vi "FPGA_Main.vi"() -> ()   [LabVIEW 2019]
uses:
  L298N_Driver/L298N_Action_Enum.ctl
  L298N_Ref_FPGA.ctl
  <vilib>/Platform/TimedLoop/XDataNode/timing_clust.ctl
  <vilib>/Platform/TimedLoop/XDataNode/nitl_modes.ctl
  <vilib>/Platform/TimedLoop/XDataNode/wakeup.ctl
  <vilib>/rvi/Emulation/niFpgaSctlEmulationGetInTimedLoop.vi
  <vilib>/rvi/Emulation/niFpgaEmulationReportErrorSimple.vi
  <vilib>/rvi/Emulation/niFpgaGetClockAttributes.vi
  <vilib>/rvi/Emulation/niFpgaCriticalErrorInLSC.vi
  <vilib>/rvi/Emulation/niFpgaProcessEmulError.vi
  <vilib>/rvi/eio/common/nirviEmuTemplateMethod_errors.vi
  <vilib>/Platform/TimedLoop/XDataNode/XDataNode.xnode
  <vilib>/eio/EIONode/EIONode.xnode
  <vilib>/Platform/TimedLoop/XDataNode/XDNodeRunTimeDep.lvlib
panel:
  out "Presence_Cabine":bool[](array[boolean])
  out "Portes_Fermees":bool[](array[boolean])
  out "Portes_Ouvertes":bool[](array[boolean])
  in  "CMD_Moteur_Porte_3":T1
  in  "CMD_Moteur_Porte_2":T1
  in  "CMD_Moteur_Porte_1":T1
  in  "CMD_Moteur_Porte_RDC":T1
  in  "STOP":bool
  in  "CMD_Moteur_Cabine":T1
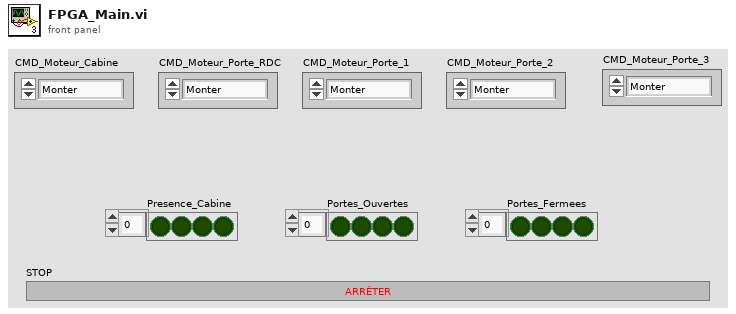
[diagram p1: front panel]
types:
  T1 = typedef "L298N_Action_Enum.ctl" = enum16{"Monter", "Descendre", "Arreter"}
  T2 = typedef "L298N_Ref_FPGA.ctl" = cluster{"Positive_Move":refnum<k21>, "Negative_Move":refnum<k21>}
  T3 = typedef "XDNodeRunTimeDep.lvlib/timing_clust.ctl" = cluster{"Expected End [f-1]":u64, "Actual End [f-1]":u64, "Finished Late? [f-1]":bool, "Expected End [i-1]":u64, "Actual End [i-1]":u64, "Finished Late? [i-1]":bool, "Expected Start [i]":u64, "Actual Start [i]":u64, "Expected Start [f]":u64, "Actual Start [f]":u64, "Source Name":string, "Structure Name":string, "Period":i64, "Deadline":i64, "Offset":i64, "Start":i64, "Priority":i32, "Timeout":i32, "Mode":T4, "Wakeup Reason":T5, "Error":errorcluster, "Source Type":string, "Secondary Source Type":string, "Global End Time":u64, "Global Start Time":u64, "Frame Duration":u64, "Iteration Duration":u64, "Assigned CPU":i32, "I/O Scan Engine Mode":u32}
  T4 = typedef "XDNodeRunTimeDep.lvlib/nitl_modes.ctl" = enum32{"No Change", "Process missed periods, maintain original phase", "Discard missed periods, maintain original phase", "Process missed periods, ignore original phase", "Discard missed periods, ignore original phase"}
  T5 = typedef "XDNodeRunTimeDep.lvlib/wakeup.ctl" = enum32{"Normal", "Aborted", "Asynchronous wakeup", "Timing source error", "Timed loop error", "Timeout"}
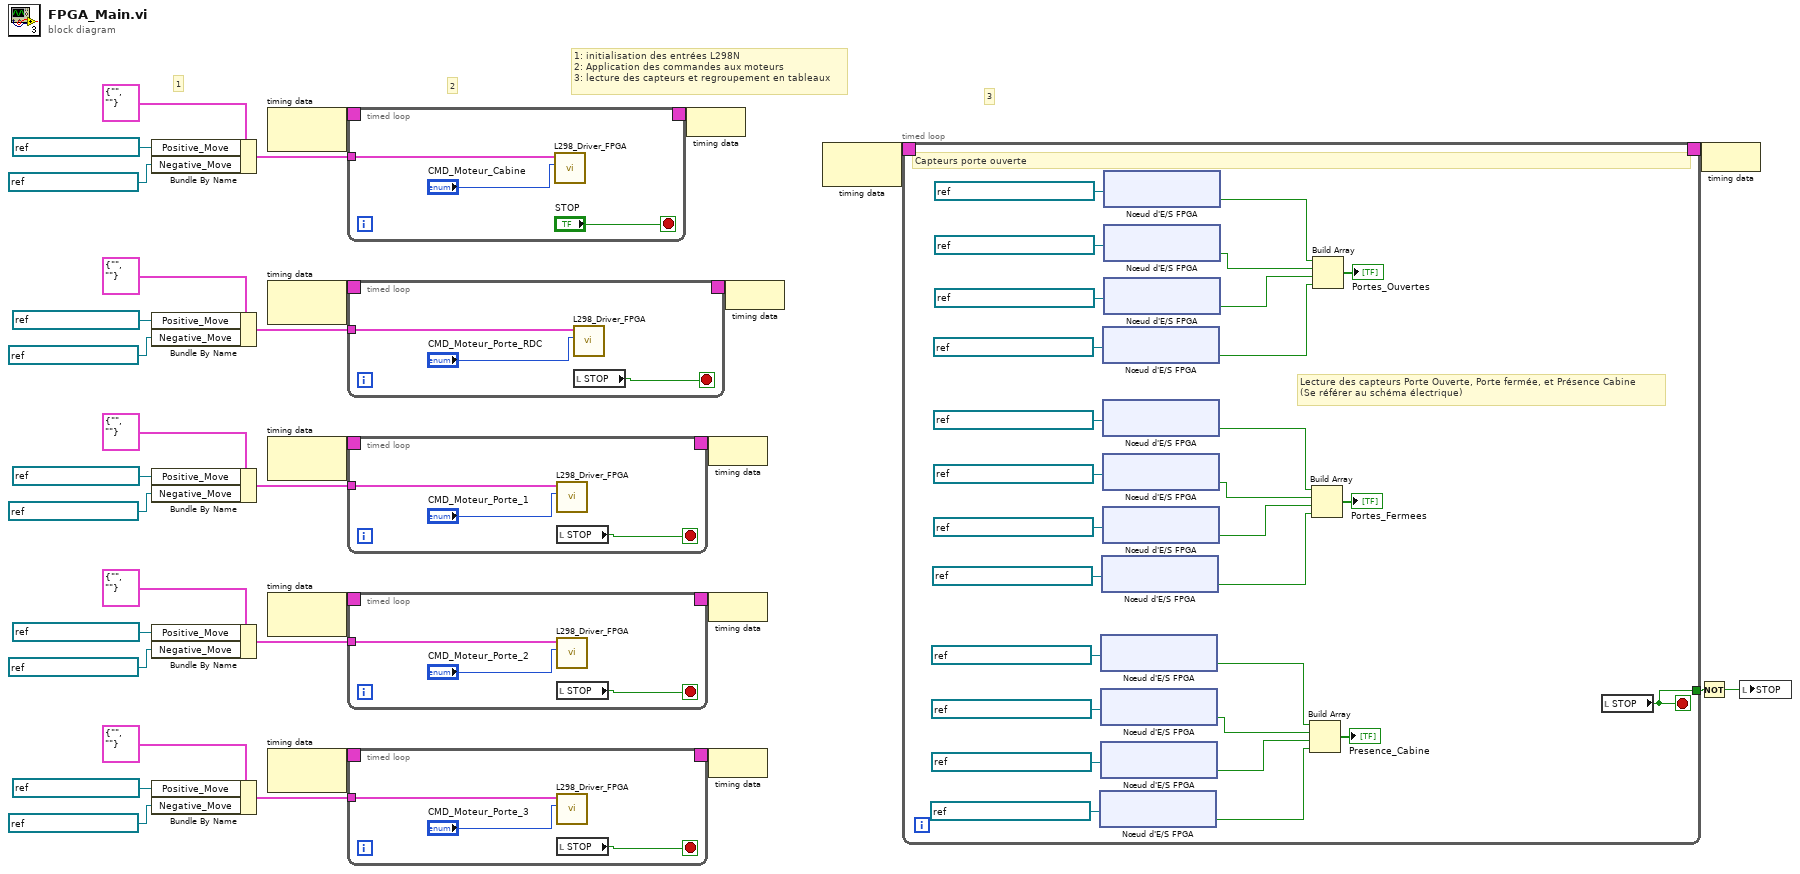
[diagram p0: block diagram]
diagram:
  # "1: initialisation des entrées L298N\n2: Application des commandes aux moteurs \n3: lecture des capteurs et regroupement en tableaux"
  # "3"
  # "2"
  # "1"
  n1 = Bundle By Name(cluster=T2 {"Positive_Move"="", "Negative_Move"=""} ("L298N_Ref_FPGA"), "Positive_Move"=refnum<k21> "ConnectorB/DIO1", "Negative_Move"=refnum<k21> "ConnectorB/DIO0") -> (w33:T2)
  n2 = Bundle By Name(cluster=T2 {"Positive_Move"="", "Negative_Move"=""} ("L298N_Ref_FPGA"), "Positive_Move"=refnum<k21> "ConnectorB/DIO2", "Negative_Move"=refnum<k21> "ConnectorB/DIO3") -> (w28:T2)
  n3 = Bundle By Name(cluster=T2 {"Positive_Move"="", "Negative_Move"=""} ("L298N_Ref_FPGA"), "Positive_Move"=refnum<k21> "ConnectorB/DIO4", "Negative_Move"=refnum<k21> "ConnectorB/DIO5") -> (w25:T2)
  n4 = Bundle By Name(cluster=T2 {"Positive_Move"="", "Negative_Move"=""} ("L298N_Ref_FPGA"), "Positive_Move"=refnum<k21> "ConnectorB/DIO6", "Negative_Move"=refnum<k21> "ConnectorB/DIO7") -> (w20:T2)
  n5 = Bundle By Name(cluster=T2 {"Positive_Move"="", "Negative_Move"=""} ("L298N_Ref_FPGA"), "Positive_Move"=refnum<k21> "ConnectorB/DIO8", "Negative_Move"=refnum<k21> "ConnectorB/DIO9") -> (w17:T2)
  n6 = node-c288() -> (w14:T3)  [unwired: 1 in]
  n7 = node-c288() -> (w12:T3)  [unwired: 1 in]
  n8 = node-c288() -> (w10:T3)  [unwired: 1 in]
  n9 = node-c288() -> (w8:T3)  [unwired: 1 in]
  n10 = node-c288() -> (w6:T3)  [unwired: 1 in]
  n11 = timed-loop {
    tunnel: w33 -> [w37]
    timing: w14 -> [_]
    timing-out: [_] -> w13
    stop <- "STOP" stop-if-true
    n12 = call "L298_Driver_FPGA.vi"("Action_Moteur"="CMD_Moteur_Cabine", "L298N_Ref_FPGA"=w37) -> ()  [unwired: 10 in]
  }
  n13 = timed-loop {
    tunnel: w28 -> [w42]
    timing: w12 -> [_]
    timing-out: [_] -> w11
    stop <- w40 stop-if-true
    n14 = call "L298_Driver_FPGA.vi"("Action_Moteur"="CMD_Moteur_Porte_RDC", "L298N_Ref_FPGA"=w42) -> ()  [unwired: 10 in]
    n15 = local read "STOP"() -> (w40:bool)
  }
  n16 = timed-loop {
    tunnel: w25 -> [w47]
    timing: w10 -> [_]
    timing-out: [_] -> w9
    stop <- w45 stop-if-true
    n17 = call "L298_Driver_FPGA.vi"("Action_Moteur"="CMD_Moteur_Porte_1", "L298N_Ref_FPGA"=w47) -> ()  [unwired: 10 in]
    n18 = local read "STOP"() -> (w45:bool)
  }
  n19 = timed-loop {
    tunnel: w20 -> [w52]
    timing: w8 -> [_]
    timing-out: [_] -> w7
    stop <- w50 stop-if-true
    n20 = call "L298_Driver_FPGA.vi"("Action_Moteur"="CMD_Moteur_Porte_2", "L298N_Ref_FPGA"=w52) -> ()  [unwired: 10 in]
    n21 = local read "STOP"() -> (w50:bool)
  }
  n22 = timed-loop {
    tunnel: w17 -> [w57]
    timing: w6 -> [_]
    timing-out: [_] -> w5
    stop <- w55 stop-if-true
    n23 = call "L298_Driver_FPGA.vi"("Action_Moteur"="CMD_Moteur_Porte_3", "L298N_Ref_FPGA"=w57) -> ()  [unwired: 10 in]
    n24 = local read "STOP"() -> (w55:bool)
  }
  n25 = node-c288(w13) -> ()
  n26 = node-c288(w9) -> ()
  n27 = node-c288(w7) -> ()
  n28 = node-c288(w5) -> ()
  n29 = node-c288(w11) -> ()
  n30 = node-c288() -> (w4:T3)  [unwired: 1 in]
  n31 = timed-loop {
    timing: w4 -> [_]
    timing-out: [_] -> w3
    tunnel: [w60] -> w2
    stop <- w60 stop-if-true
    # "Lecture des capteurs Porte Ouverte, Porte fermée, et Présence Cabine\n(Se référer au schéma électrique)"
    # "Capteurs porte ouverte"
    n32 = xnode "Nœud d'E/S FPGA"("E/S FPGA en entrée"=refnum<k21> "ConnectorA/DIO11") -> ("Élément d'E/S"=w64:bool)  [unwired: 1 out]
    n33 = xnode "Nœud d'E/S FPGA"("E/S FPGA en entrée"=refnum<k21> "ConnectorA/DIO0") -> ("Élément d'E/S"=w65:bool)  [unwired: 1 out]
    n34 = xnode "Nœud d'E/S FPGA"("E/S FPGA en entrée"=refnum<k21> "ConnectorA/DIO5") -> ("Élément d'E/S"=w62:bool)  [unwired: 1 out]
    n35 = xnode "Nœud d'E/S FPGA"("E/S FPGA en entrée"=refnum<k21> "ConnectorA/DIO6") -> ("Élément d'E/S"=w63:bool)  [unwired: 1 out]
    n36 = xnode "Nœud d'E/S FPGA"("E/S FPGA en entrée"=refnum<k21> "ConnectorA/DIO10") -> ("Élément d'E/S"=w75:bool)  [unwired: 1 out]
    n37 = xnode "Nœud d'E/S FPGA"("E/S FPGA en entrée"=refnum<k21> "ConnectorA/DIO8") -> ("Élément d'E/S"=w82:bool)  [unwired: 1 out]
    n38 = xnode "Nœud d'E/S FPGA"("E/S FPGA en entrée"=refnum<k21> "ConnectorA/DIO1") -> ("Élément d'E/S"=w74:bool)  [unwired: 1 out]
    n39 = xnode "Nœud d'E/S FPGA"("E/S FPGA en entrée"=refnum<k21> "ConnectorA/DIO4") -> ("Élément d'E/S"=w77:bool)  [unwired: 1 out]
    n40 = xnode "Nœud d'E/S FPGA"("E/S FPGA en entrée"=refnum<k21> "ConnectorA/DIO9") -> ("Élément d'E/S"=w76:bool)  [unwired: 1 out]
    n41 = xnode "Nœud d'E/S FPGA"("E/S FPGA en entrée"=refnum<k21> "ConnectorA/DIO3") -> ("Élément d'E/S"=w83:bool)  [unwired: 1 out]
    n42 = xnode "Nœud d'E/S FPGA"("E/S FPGA en entrée"=refnum<k21> "ConnectorA/DIO2") -> ("Élément d'E/S"=w80:bool)  [unwired: 1 out]
    n43 = xnode "Nœud d'E/S FPGA"("E/S FPGA en entrée"=refnum<k21> "ConnectorA/DIO7") -> ("Élément d'E/S"=w81:bool)  [unwired: 1 out]
    n44 = Build Array(w65, w62, w63, w64) -> (→"Presence_Cabine":bool[])
    n45 = Build Array(w74, w77, w76, w75) -> (→"Portes_Fermees":bool[])
    n46 = Build Array(w83, w80, w81, w82) -> (→"Portes_Ouvertes":bool[])
    n47 = local read "STOP"() -> (w60:bool)
  }
  n48 = Not(x=w2) -> (.not. x?=w1:bool)
  n49 = node-c288(w3) -> ()
  n50 = local write "STOP"(w1) -> ()
